vi "set_iterations_per_pixel.vi"(8 "error in (no error)":errorcluster, 10 "iterations per pixel":i32, 11 "FPGAWrapperDL090211Galvo in":refnum<class "FPGAWrapperDL090211Galvo.lvclass">) -> (0 "error out":errorcluster, 3 "FPGAWrapperDL090211Galvo out":refnum<class "FPGAWrapperDL090211Galvo.lvclass">)   [LabVIEW 2010, in "FPGAWrapperDL090211Galvo.lvclass"]
uses:
  FPGAWrapperDL090211Galvo.lvclass
  <vilib>/rvi/interface/nirviReadWriteControl/nirviReadWriteControl.xnode
  FPGA_VI_ref.ctl
  <vilib>/rvi/interface/common/niFpgaNodeNameForErrorReporting.ctl
  <vilib>/rvi/errors/niLvFpgaWhatHappensToTopLevelVI.ctl
  <vilib>/Utility/error.llb/Error Cluster From Error Code.vi
  <vilib>/rvi/errors/niLvFpgaAdjustHostInterfaceError.vi
  NiFpgaLv.dll
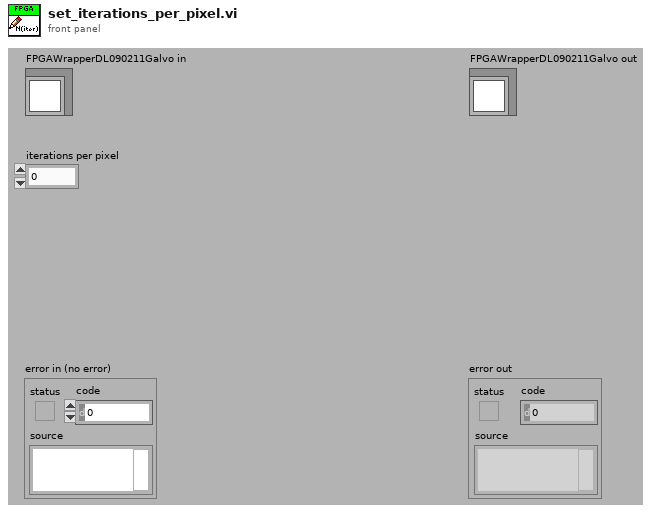
[diagram p1: front panel]
types:
  T1 = typedef "niFpgaNodeNameForErrorReporting.ctl" = enum16{"Open FPGA VI Reference", "Read/Write Control", "Invoke Method: Abort", "Invoke Method: Acknowledge IRQ", "Invoke Method: Download", "Invoke Method: FIFO.Configure", "Invoke Method: FIFO.Read", "Invoke Method: FIFO.Start", "Invoke Method: FIFO.Stop", "Invoke Method: FIFO.Write", "Invoke Method: Reset", "Invoke Method: Run", "Invoke Method: Wait on IRQ", "Close FPGA VI Reference"}
  T2 = typedef "niLvFpgaWhatHappensToTopLevelVI.ctl" = enum16{"top level VI scripted behind XNode", "top level VI inlined behind XNode"}
  T3 = typedef "FPGAWrapperDL090211Galvo.lvclass/FPGA_VI_ref.ctl" = refnum<k20>
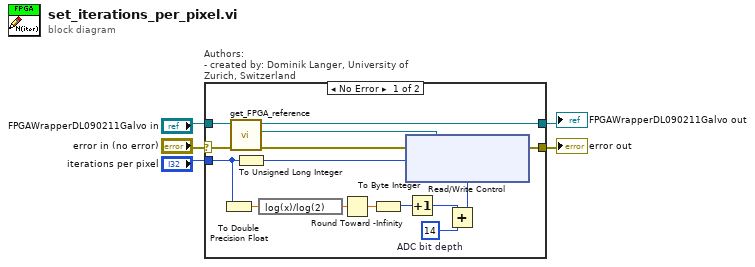
[diagram p0: block diagram]
diagram:
  n1 = case "Authors: \n- created by: Dominik Langer, University of Zurich, Switzerland" shown="No Error" "error in (no error)" {
    selector: "error in (no error)" -> [w15 w80]
    tunnel: "FPGAWrapperDL090211Galvo in" -> [w20 w81]
    tunnel: [w19 w81] -> w1
    tunnel: [w16 w80] -> w2
    tunnel: "iterations per pixel" -> [w6 _]
    frame No Error {
      w12 = i8 14  # ADC bit depth
      n2 = To Double Precision Float(number=w6) -> (double precision float=w8:dbl)
      n3 = call-dynamic "get_FPGA_reference.vi"("error in (no error)"=w15, "FPGAWrapperDL090211Galvo in"=w20) -> ("error out"=w18:errorcluster, "FPGA VI reference"=w17:T3, "FPGAWrapperDL090211Galvo out"=w19:refnum<class "FPGAWrapperDL090211Galvo.lvclass">)  [unwired: 6 in, 1 out]
      n4 = To Unsigned Long Integer(number=w6) -> (unsigned 32bit integer=w14:u32)
      n5 = expression code="log(x)/log(2)"(w8) -> (w7:dbl)
      n6 = Round Toward -Infinity(1:w7) -> (0:w13:dbl)
      n7 = To Byte Integer(number=w13) -> (8bit integer=w11:i8)
      n8 = Increment(x=w11) -> (x+1=w10:i8)
      n9 = Add(x=w10, y=w12) -> (x+y=w9:i8)
      n10 = xnode "Read/Write Control"("FPGA VI Reference In"=w17, "error in"=w18, "iterations per pixel"=w14, "maximum bit depth"=w9) -> ("error out"=w16:errorcluster)  [unwired: 1 out]
    }
    frame Error {
    }
  }
  "error out" <- w2
  "FPGAWrapperDL090211Galvo out" <- w1
